vi "Tag Field.vi"() -> (3 "Tag Field":string)   [LabVIEW 2016]
doc: "Assign <B>Tag: <tag></B> to <B>Tag Field</B>"
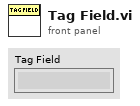
[diagram p1: front panel]
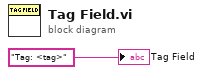
[diagram p0: block diagram]
diagram:
  "Tag Field" <- "Tag: <tag>"
